vi "Read object configuration.vi"(6 "Object name":string, 8 "Error In":errorcluster, 9 "type":variant, 10 "File path":path, 11 "object":refnum<class>) -> (0 "Error Out":errorcluster, 1 "Configuration":variant, 2 "File path out":path, 4 "Section out":string, 5 "found?":bool)   [LabVIEW 2016]
uses:
  <vilib>/Utility/config.llb/NI_LVConfig.lvlib
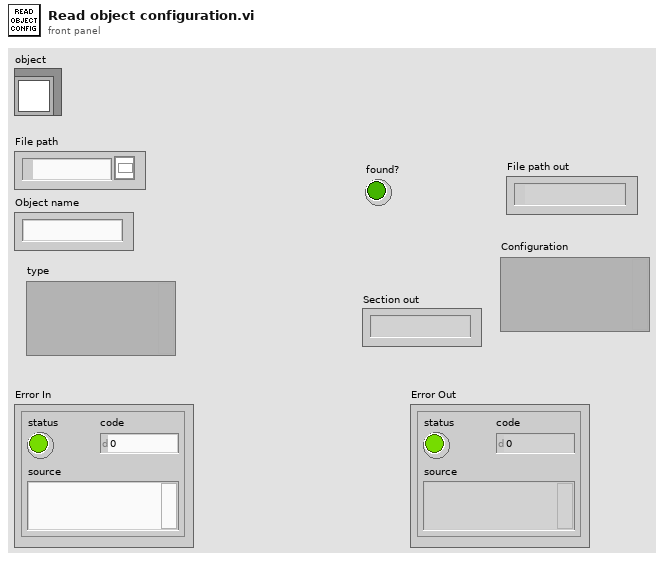
[diagram p1: front panel]
types:
  T1 = typedef "NI_LVConfig.lvlib/Config Data RefNum.ctl" = refnum<k1>
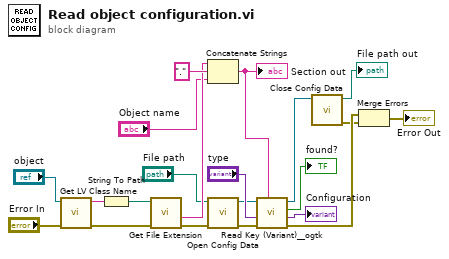
[diagram p0: block diagram]
diagram:
  n1 = call <vilib>:"Get LV Class Name.vi"("error in (no error)"="Error In", "object"="object") -> ("error out"=w18:errorcluster, "class name"=w20:string)  [unwired: 8 in]
  n2 = String To Path(string=w20) -> (path=w16:path)
  n3 = call <vilib>:"Get File Extension.vi"("error in (no error)"=w18, "file"=w16) -> ("error out"=w19:errorcluster, "filename without extension"=w17:string)  [unwired: 5 in, 3 out]
  n4 = Concatenate Strings(w17, "." ("string"), "Object name") -> (w2:string)
  "Section out" <- w2
  n5 = call <vilib>:"Open Config Data.vi"("error in (no error)"=w19, "configuration file path"="File path") -> ("error out"=w10:errorcluster, "refnum"=w11:T1)  [unwired: 7 in, 1 out]
  n6 = call <userlib>:"Read Key (Variant)__ogtk.vi"("section"=w2, "error in (no error)"=w10, "type"="type", "refnum"=w11) -> ("error out"=w8:errorcluster, "key-value"=→"Configuration":variant, "found?"=→"found?":bool, "refnum out"=w9:T1)  [unwired: 4 in]
  n7 = call <vilib>:"Close Config Data.vi"("refnum"=w9) -> ("error out"=w7:errorcluster, "file path"=→"File path out":path)  [unwired: 9 in]
  n8 = Merge Errors(w8, w7) -> (→"Error Out":errorcluster)
